vi "Get JoyStick Values.vi"(11 "Joystick Name":string="My Joystick RefNum") -> (2 "Buttons":bool[](array[boolean]), 3 "Axes":dbl[](array[numeric]))   [LabVIEW 2014]
doc: "Writes joystick values to a the dashboard."
uses:
  <vilib>/Rock Robotics/WPI/Joystick/WPI_JoystickGetSetRefNum.vi
  <vilib>/Rock Robotics/Network Tables/SD Write Boolean Array.vi
  <vilib>/Rock Robotics/Network Tables/SD Write Numeric Array.vi
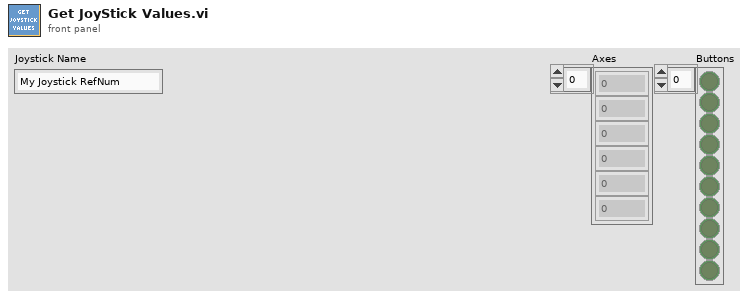
[diagram p1: front panel]
types:
  T1 = typedef "WPI_JoystickDevRef.ctl" = cluster{"Device":T2}
  T2 = typedef "WPI_JoystickDeviceEnum.ctl" = enum16{"USB 0", "USB 1", "USB 2", "USB 3", "USB 4", "USB 5"}
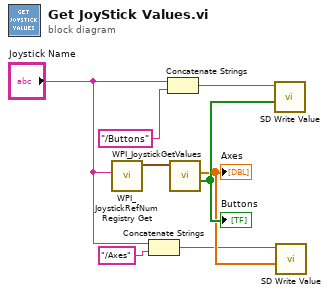
[diagram p0: block diagram]
diagram:
  n1 = call <vilib>:"WPI_JoystickRefNum Registry Get.vi"("refnum name"="Joystick Name") -> ("JoystickDevRef"=w8:T1)  [unwired: 1 in, 9 out]
  n2 = Concatenate Strings("Joystick Name", "/Axes" ("Name")) -> (w1:string)
  n3 = Concatenate Strings("Joystick Name", "/Buttons" ("Name")) -> (w2:string)
  n4 = call <vilib>:"WPI_JoystickGetValues.vi"("JoystickDevRef"=w8) -> ("Buttons"=w7:bool[], "Axes"=w6:dbl[])  [unwired: 6 in, 3 out]
  "Axes" <- w6
  "Buttons" <- w7
  n5 = call-poly <vilib>:"SD Write Value.vi"("Boolean Array"=w7, "Name"=w2) -> ()  [unwired: 8 in, 2 out]
  n6 = call-poly <vilib>:"SD Write Value.vi"("Numeric Array"=w6, "Name"=w1) -> ()  [unwired: 8 in, 2 out]
